vi "User Event Abort.vi"(7 "Enum":enum16{"Create", "Destroy", "Get"}(ring), 8 "error in (no error)":errorcluster) -> (0 "error out":errorcluster, 3 "User Event Out":refnum<user-event>)   [LabVIEW 2020, in "Architecture Support.lvlib"]
uses:
  Architecture Support.lvlib
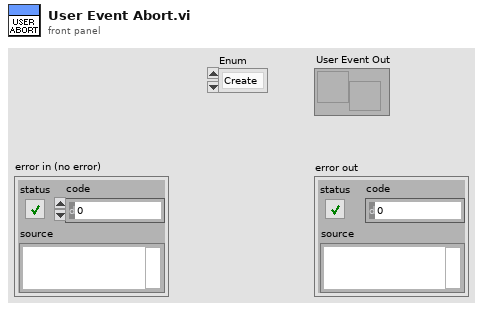
[diagram p1: front panel]
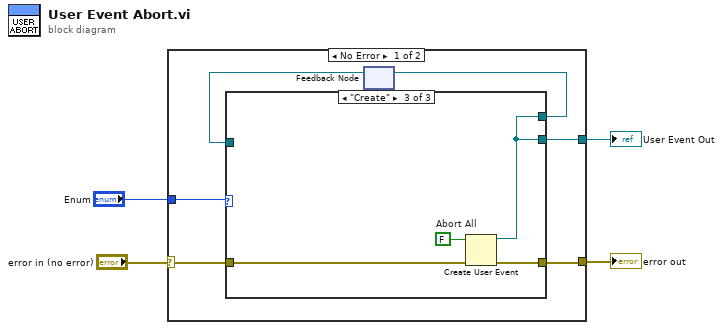
[diagram p0: block diagram]
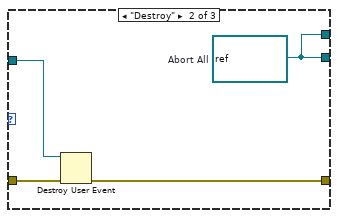
[diagram p3: hidden frame]
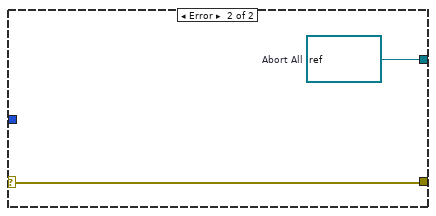
[diagram p4: hidden frame]
diagram:
  n1 = case shown="No Error" "error in (no error)" {
    selector: "error in (no error)" -> [w9 w21]
    tunnel: "Enum" -> [w10 _]
    tunnel: [w8 w22] -> w1
    tunnel: [w5 w21] -> w2
    frame No Error {
      n2 = feedback #1() -> (w6:refnum<user-event>)  [unwired: 1 in]
      n3 = case shown="\"Create\"" w10 {
        tunnel: w9 -> [w12 w16 w20]
        tunnel: [w11 w13 w18] -> w8
        tunnel: w6 -> [w11 w15 _]
        tunnel: [w11 w13 w18] -> w7
        tunnel: [w12 w14 w17] -> w5
        frame "Get", Default {
        }
        frame "Destroy" {
          w13 = refnum<user-event> refnum  # Abort All
          n4 = Destroy User Event(user event=w15, error in=w16) -> (error out=w14:errorcluster)
        }
        frame "Create" {
          w19 = FALSE  # Abort All
          n5 = Create User Event(user event datatype=w19, error in=w20) -> (user event=w18:refnum<user-event>, error out=w17:errorcluster)
        }
      }
      n6 = feedback-in #1(w7) -> ()
    }
    frame Error {
      w22 = refnum<user-event> refnum  # Abort All
    }
  }
  "error out" <- w2
  "User Event Out" <- w1
